vi "ASI Get Num Of Controls.vi"(10 "piNumberOfControls":i32, 11 "iCameraID":i32) -> (2 "piNumberOfControls out":i32, 3 "function return":i32)   [LabVIEW 2023, in "ASICamera2_no_err.lvlib"]
doc: "ASICAMERA_API ASI_ERROR_CODE ASIGetNumOfControls(int iCameraID, int * piNumberOfControls);"
uses:
  ASICamera2_no_err.lvlib
  ASICamera2.dll
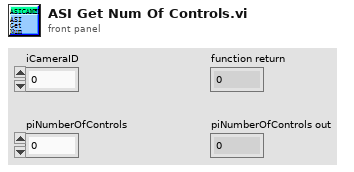
[diagram p1: front panel]
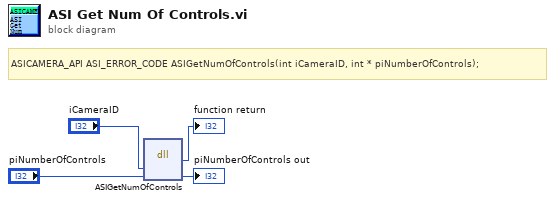
[diagram p0: block diagram]
diagram:
  # "ASICAMERA_API ASI_ERROR_CODE ASIGetNumOfControls(int iCameraID, int * piNumberOfControls);"
  n1 = dll-call lib="C:/Users/quantum/Documents/LVDAQ/ConcreteClasses/ConcreteInstrumentClasses/CameraClasses/ZWO_ASI_LV/Labview_ASI_demo_64bit_221128/user.lib/ASICamera2_no_err/ASICamera2.*" fn="ASIGetNumOfControls"("iCameraID"="iCameraID", "piNumberOfControls"="piNumberOfControls") -> (→"function return":i32, "piNumberOfControls"=→"piNumberOfControls out":i32)  [unwired: 4 in, 2 out]
